vi "Main Loop.vi"(8 "error in (no error)":errorcluster, 10 "Chart Notifier":refnum<notifier>, 11 "Message Queues":T7) -> (0 "error out":errorcluster)   [LabVIEW 2018, in "D-O Module.lvlib" / "D-O Module Engine.lvlib"]
uses:
  D-O Module Engine.lvlib
  All Message Queues.ctl
  support/Message Queue/Message Cluster.ctl
  State Cluster.ctl
  State Enum.ctl
  Valve Clusters.ctl
  D-O Module Settings Cluster.ctl
  D-O Device Settings Cluster.ctl
  VICI Electronic Actuator/VICI Electronic Actuator Settings.ctl
  D-O Module Display.ctl
  <vilib>/Platform/TimedLoop/XDataNode/timing_clust.ctl
  <vilib>/Platform/TimedLoop/XDataNode/nitl_modes.ctl
  <vilib>/Platform/TimedLoop/XDataNode/wakeup.ctl
  Tag VIs/Tag FGV Operation Enum.ctl
  support/Message Queue/Enqueue Message (Single).vi
  <vilib>/Platform/TimedLoop/XDataNode/XDataNode.xnode
  support/Message Queue/Message Queue.lvlib
  <vilib>/Platform/TimedLoop/XDataNode/XDNodeRunTimeDep.lvlib
  D-O Module.lvlib
  Shared Variables/Dynamic Shared Variables.lvlib
  support/Command Log VIs/Command Logging.lvlib
  DIO Valve/VICI Electronic Actuator.lvlib
  support/Support Library.lvlib
panel:
  out "D-O Settings.Output Channel Names":string[](array[string])
  in  "?":T1={"State"=enum."Idle", "Start Time"=timestamp(0 s since 1904-01-01), "Current Time"=timestamp(0 s since 1904-01-01), "First Iteration"=FALSE, "Process Name"="", "Output Error"=FALSE, "Log Started"=FALSE, "Cycle Period"=50.0, "Configuration"={"Valve Settings"={"D-O Settings"={"DAQmx Task Name"="", "Output Channel"=0, "Output Channel Names"=[]}, "VICI Electronic Actuator"={"VISA resource name"="", "Mode"=enum."Two Positions With Stops", "Simulated"=FALSE}}, "Valve Type"=enum."Digital Output Valve", "Time On (Sec)"=0.0, "Time Off (Sec)"=0.0, "Run?"=FALSE}, "Data"={"D-O State"=enum."Off"}} {"Configuration"."Valve Settings"."D-O Settings"."Output Channel" items=["Choose a Channel"]}
  out "Period (s)":dbl format="%_4g"
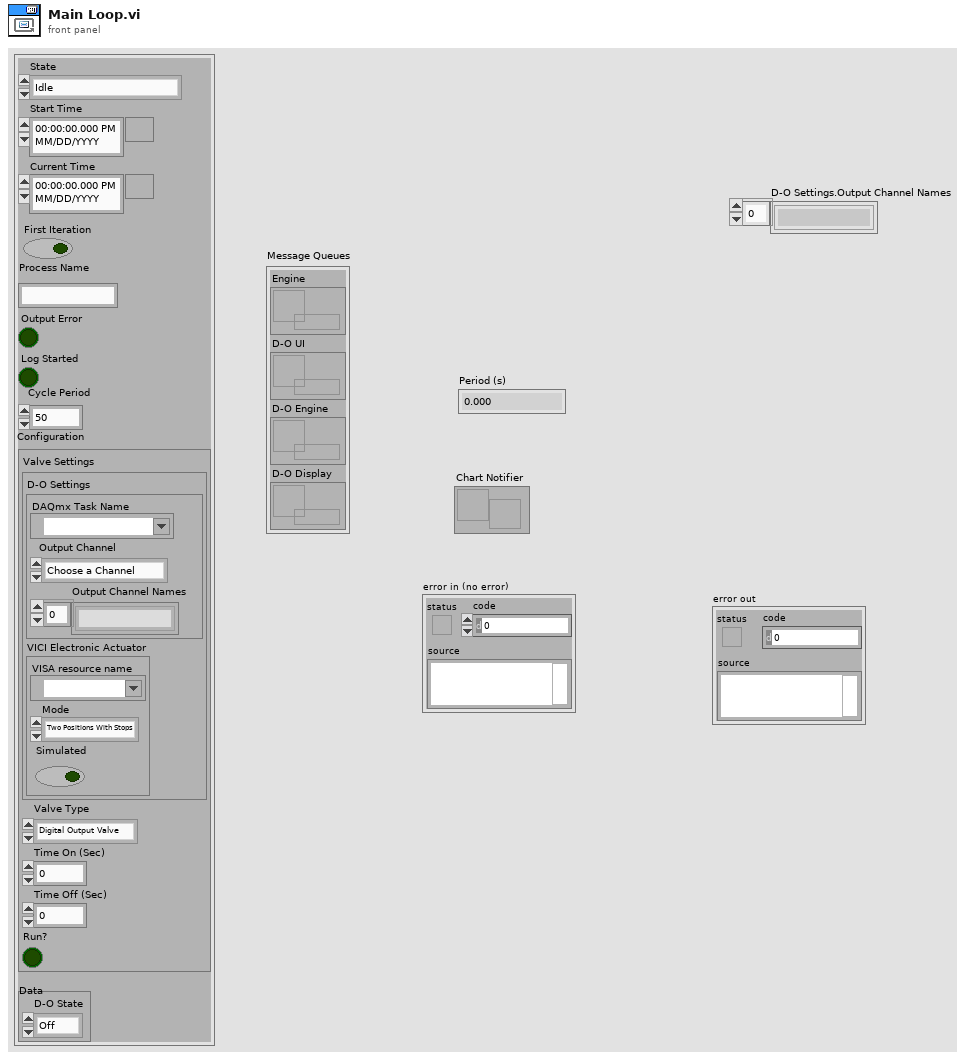
[diagram p1: front panel]
types:
  T1 = typedef "D-O Module.lvlib/D-O Module Engine.lvlib/State Cluster.ctl" = cluster{"State":T2, "Start Time":timestamp, "Current Time":timestamp, "First Iteration":bool, "Process Name":string, "Output Error":bool, "Log Started":bool, "Cycle Period":dbl, "Configuration":T3, "Data":cluster{"D-O State":enum16{"Off", "On", "Not Initialized"}}}
  T2 = typedef "D-O Module.lvlib/D-O Module Engine.lvlib/State Enum.ctl" = enum16{"Measuring", "Idle", "Paused"}
  T3 = typedef "D-O Module.lvlib/Valve Clusters.ctl" = cluster{"Valve Settings":T4, "Valve Type":enum16{"Default", "Digital Output Valve", "VICI Electronic Actuator"}, "Time On (Sec)":dbl, "Time Off (Sec)":dbl, "Run?":bool}
  T4 = typedef "D-O Module.lvlib/D-O Module Settings Cluster.ctl" = cluster{"D-O Settings":T5, "VICI Electronic Actuator":T6}
  T5 = typedef "D-O Module.lvlib/D-O Device Settings Cluster.ctl" = cluster{"DAQmx Task Name":refnum<k21>, "Output Channel":u16, "Output Channel Names":string[]}
  T6 = typedef "VICI Electronic Actuator.lvlib/VICI Electronic Actuator Settings.ctl" = cluster{"VISA resource name":refnum<visa-resource-name>, "Mode":enum16{"Two Positions With Stops", "Two Positions Without Stops", "Mutiposition"}, "Simulated":bool}
  T7 = typedef "D-O Module.lvlib/All Message Queues.ctl" = cluster{"Engine":refnum<queue>, "D-O UI":refnum<queue>, "D-O Engine":refnum<queue>, "D-O Display":refnum<queue>}
  T8 = typedef "D-O Module.lvlib/D-O Module Display.ctl" = cluster{"D-O State ":u16, "Cycle Period":dbl}
  T9 = typedef "XDNodeRunTimeDep.lvlib/timing_clust.ctl" = cluster{"Expected End [f-1]":u64, "Actual End [f-1]":u64, "Finished Late? [f-1]":bool, "Expected End [i-1]":u64, "Actual End [i-1]":u64, "Finished Late? [i-1]":bool, "Expected Start [i]":u64, "Actual Start [i]":u64, "Expected Start [f]":u64, "Actual Start [f]":u64, "Source Name":string, "Structure Name":string, "Period":i64, "Deadline":i64, "Offset":i64, "Start":i64, "Priority":i32, "Timeout":i32, "Mode":T10, "Wakeup Reason":T11, "Error":errorcluster, "Source Type":string, "Secondary Source Type":string, "Global End Time":u64, "Global Start Time":u64, "Frame Duration":u64, "Iteration Duration":u64, "Assigned CPU":i32, "I/O Scan Engine Mode":u32}
  T10 = typedef "XDNodeRunTimeDep.lvlib/nitl_modes.ctl" = enum32{"No Change", "Process missed periods, maintain original phase", "Discard missed periods, maintain original phase", "Process missed periods, ignore original phase", "Discard missed periods, ignore original phase"}
  T11 = typedef "XDNodeRunTimeDep.lvlib/wakeup.ctl" = enum32{"Normal", "Aborted", "Asynchronous wakeup", "Timing source error", "Timed loop error", "Timeout"}
  T12 = cluster{"enable? (F)":bool, "name":string, "alarm on":bool, "priority":u32, "ack type":enum16{"Auto", "User", "None", "Each Occurrence"}, "area":string, "description":string, "log? (T)":bool}
  T13 = typedef "Tag FGV Operation Enum.ctl" = enum16{"Init", "Set Notification Queue", "Create Tag", "Commit", "Write Tag (Numeric)", "Write Tag (Boolean)", "Read All Tags", "Read One Tag", "Delete Tag Category", "Set Alarm Parameters (Numeric)", "Set Alarm Parameters (Boolean)", "Enable All Alarms", "Disable All Alarms", "Delete All Tags", "Read Alarms", "Ack Alarm", "Read Alarm Parameters (Numeric)", "Read Alarm Parameters (Boolean)"}
  T14 = enum32{"u32BitField", "bool", "double", "string", "int8", "uint8", "int16", "uint16", "int32", "uint32", "int64", "uint64", "single", "double waveform", "int16 waveform", "array of boolean", "array of int8", "array of uint8", "array of int16", "array of uint16", "array of int32", "array of uint32", "array of int64", "array of uint64", "array of single", "array of double", "array of double waveform", "array of int16 waveform", "array of string", "variant", "timestamp", "fixed point", "custom"}
  T15 = enum16{"Default", "Digital Output Valve", "VICI Electronic Actuator"}
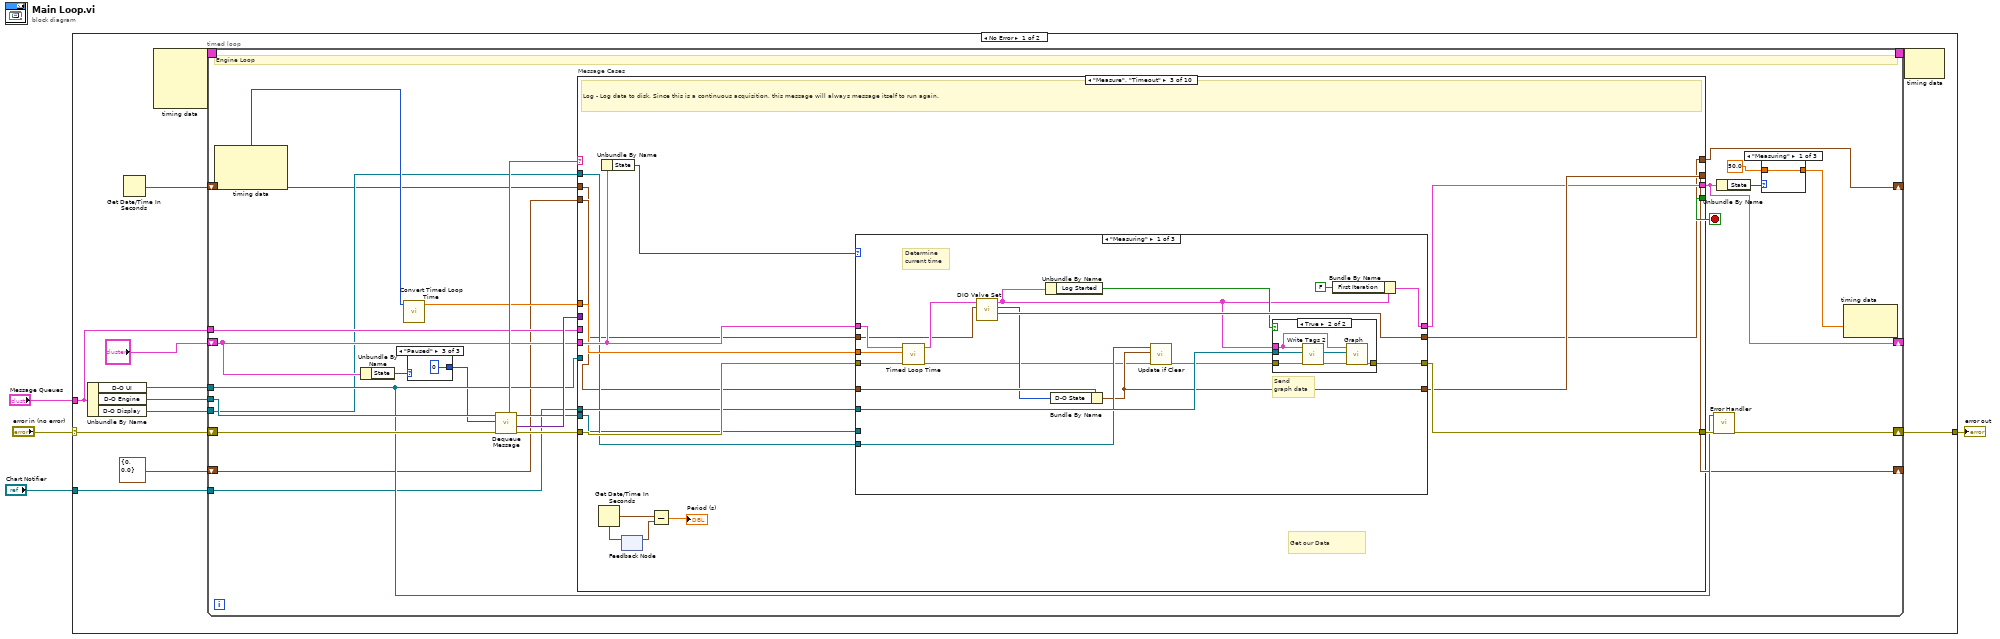
[diagram p0: block diagram]
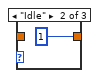
[diagram p2: hidden frame]
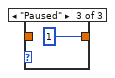
[diagram p3: hidden frame]
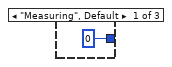
[diagram p4: hidden frame]
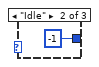
[diagram p5: hidden frame]
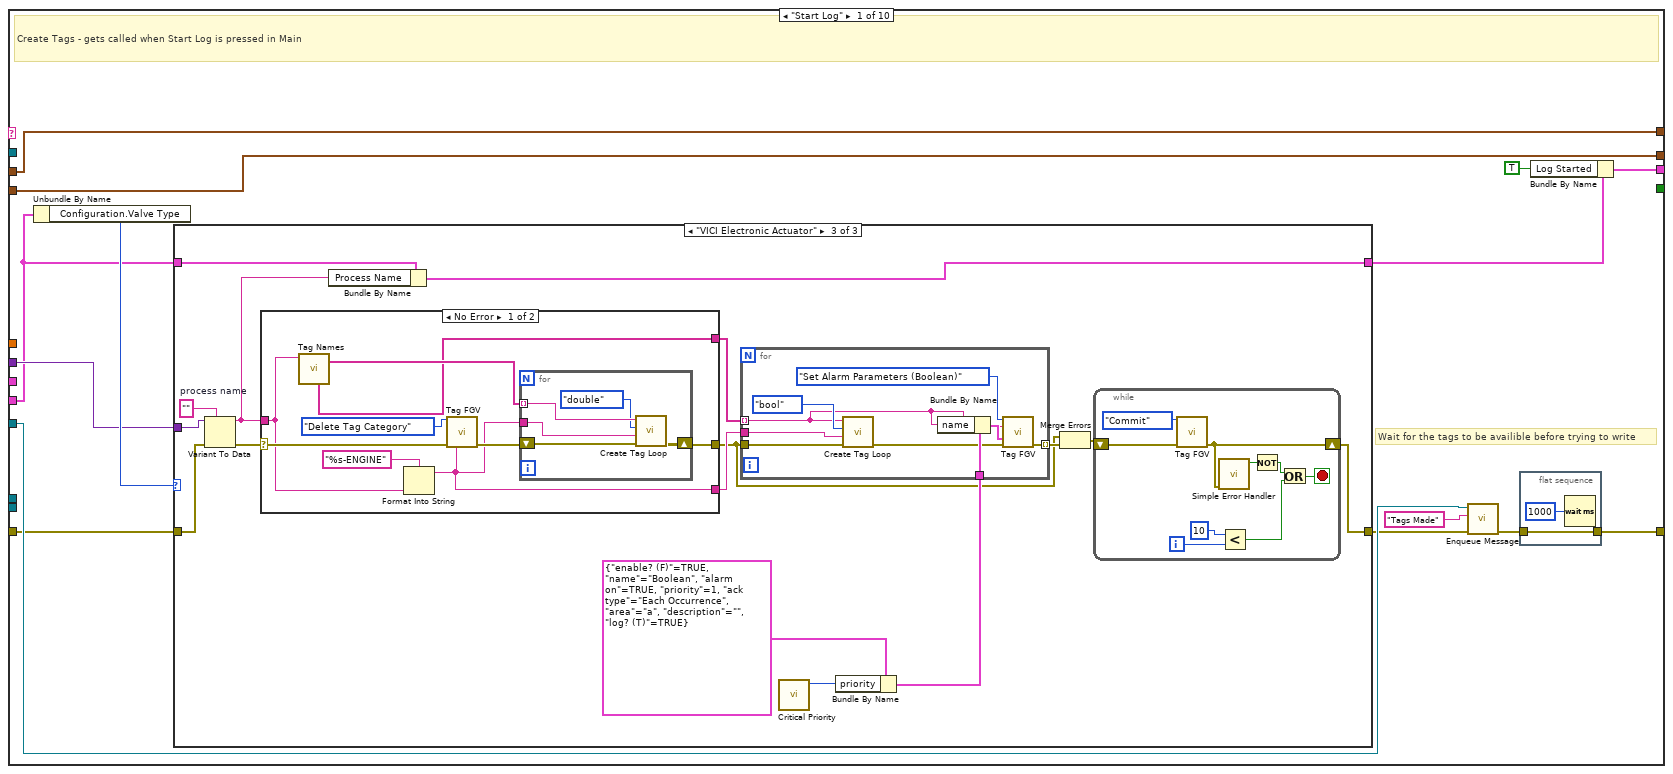
[diagram p6: hidden frame]
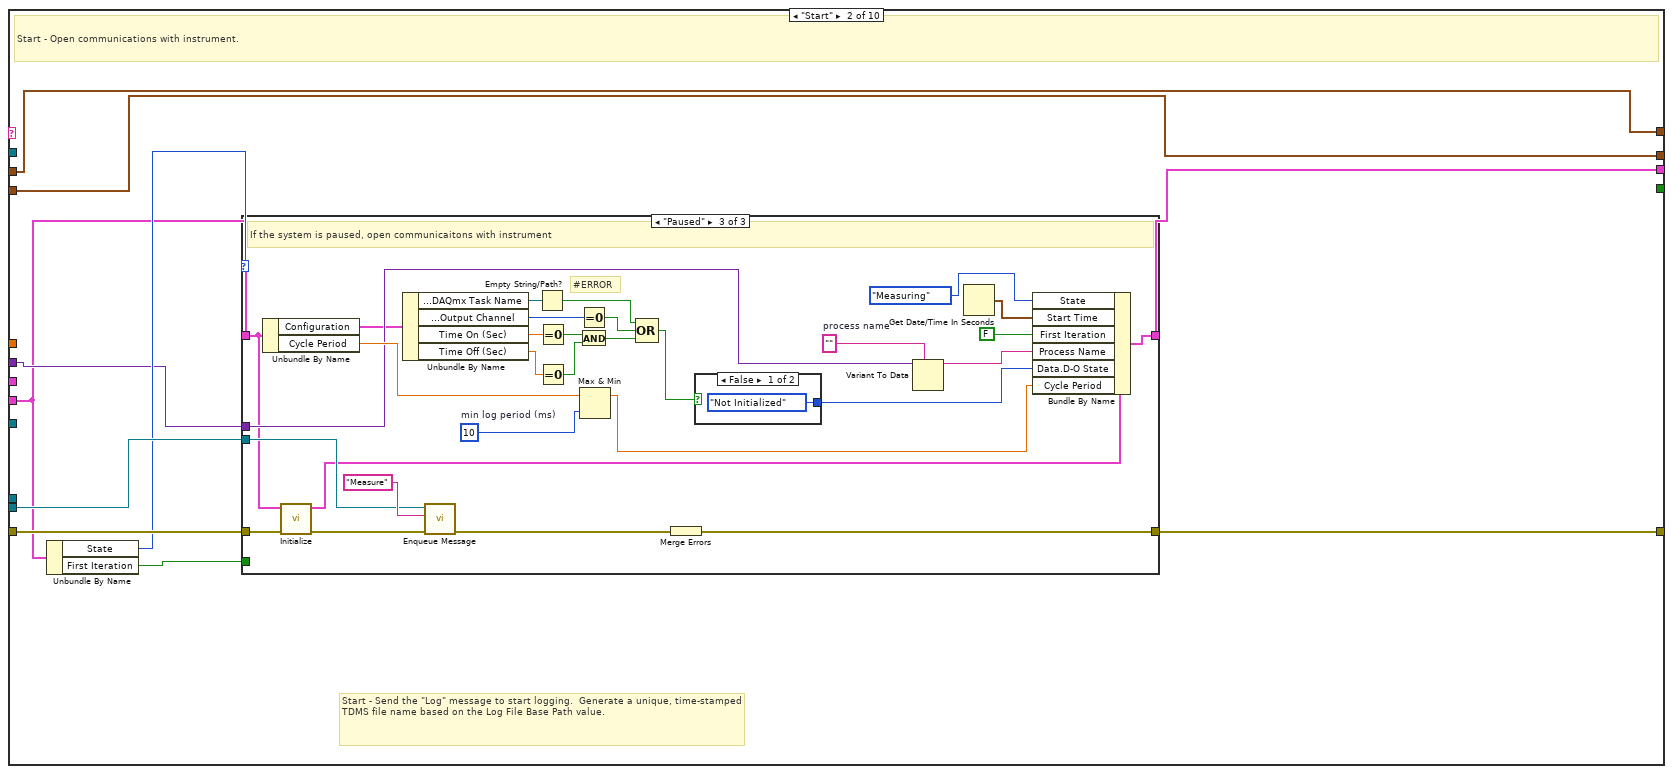
[diagram p10: hidden frame]
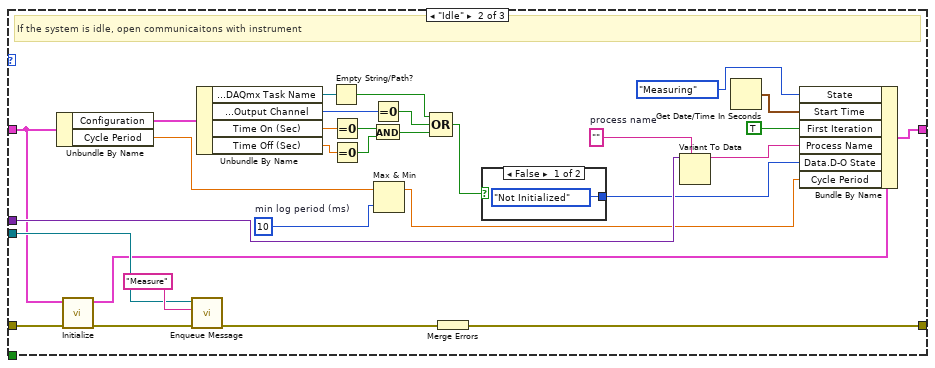
[diagram p12: hidden frame]
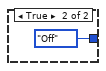
[diagram p13: hidden frame]
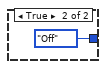
[diagram p14: hidden frame]
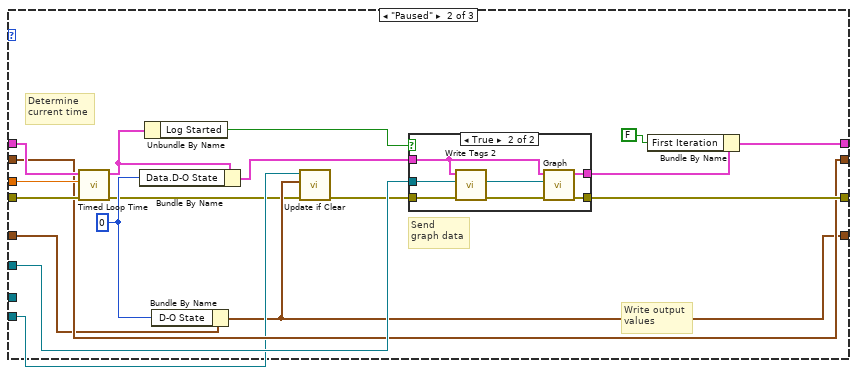
[diagram p16: hidden frame]
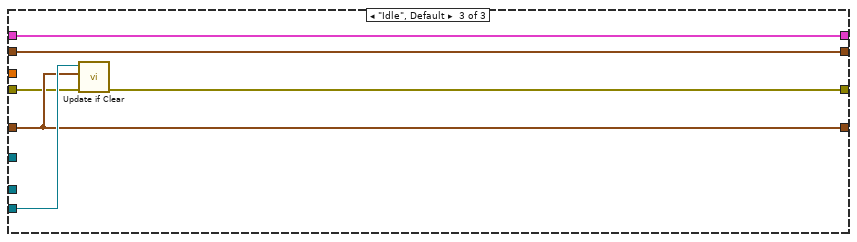
[diagram p18: hidden frame]
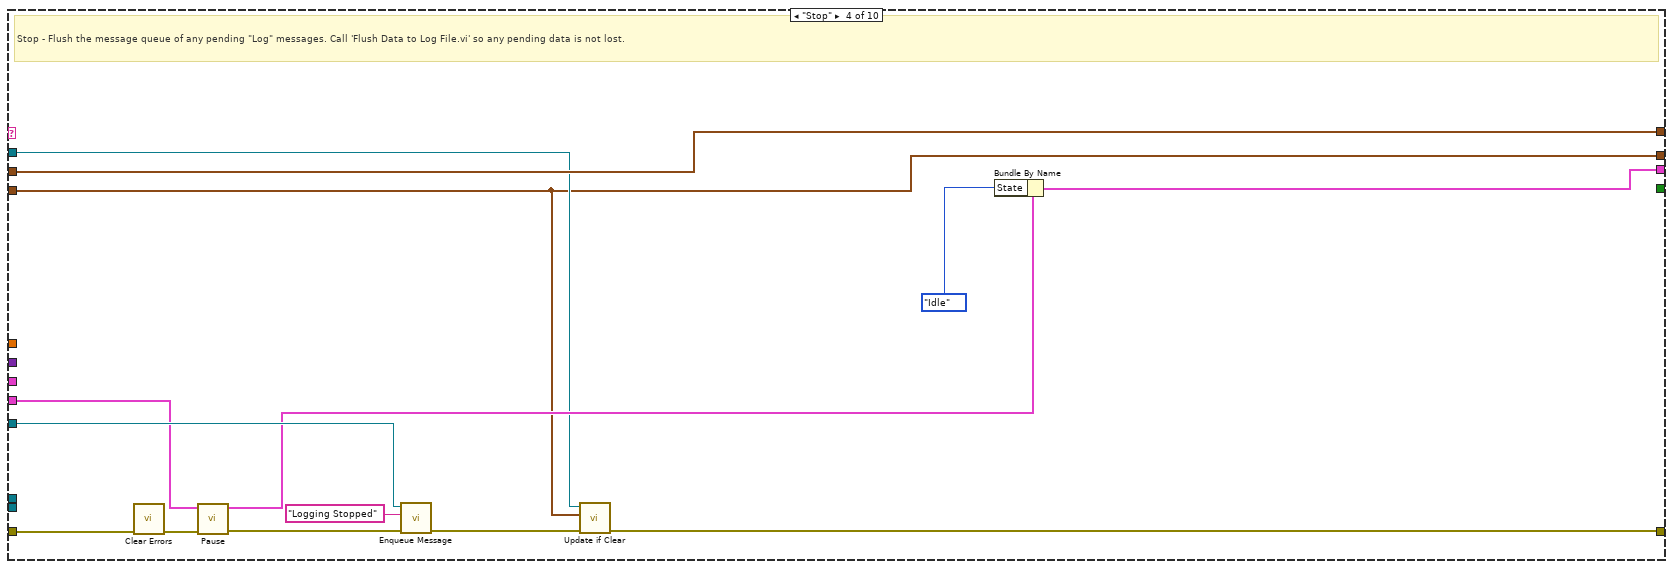
[diagram p19: hidden frame]
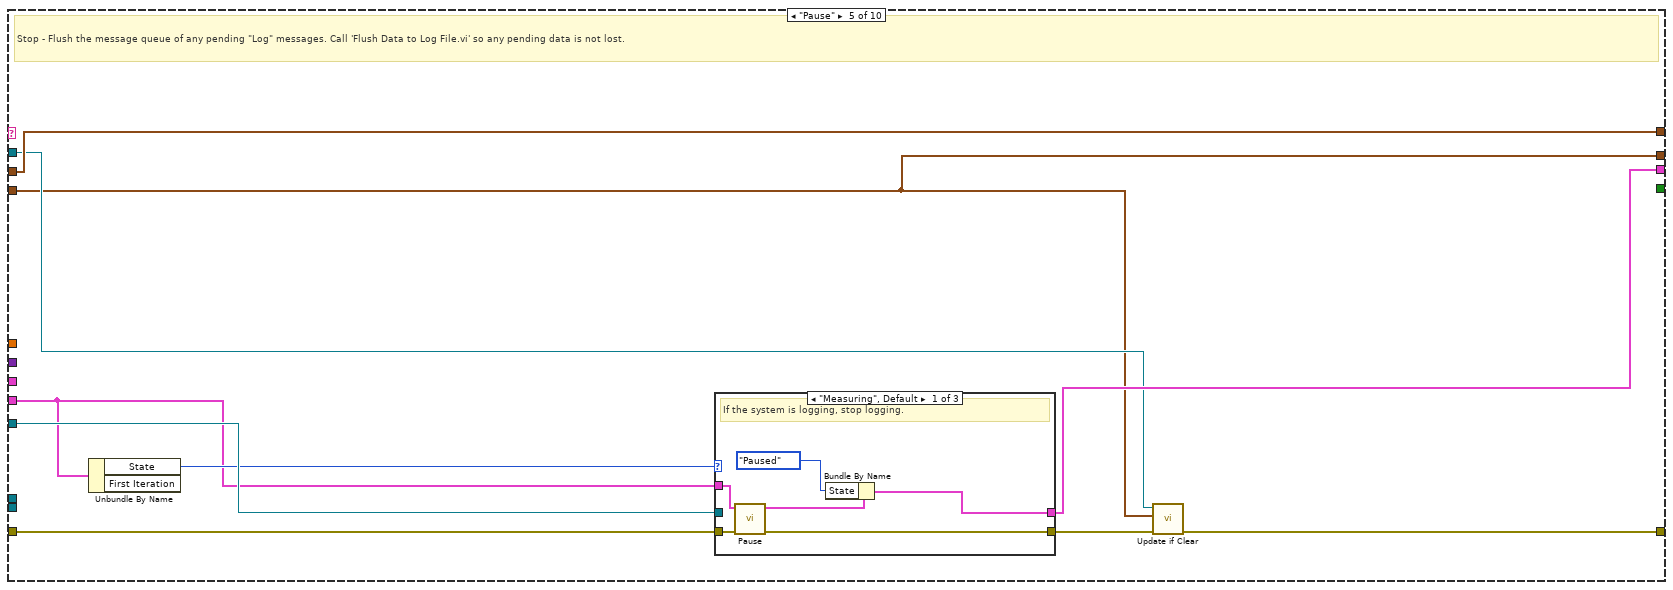
[diagram p20: hidden frame]
diagram:
  n1 = case shown="No Error" "error in (no error)" {
    selector: "error in (no error)" -> [w15 w357]
    tunnel: "Message Queues" -> [w11 _]
    tunnel: [w16 w357] -> w3
    tunnel: "Chart Notifier" -> [w9 _]
    frame No Error {
      n2 = Unbundle By Name(w11) -> ("D-O UI"=w14:refnum<queue>, "D-O Engine"=w10:refnum<queue>, "D-O Display"=w8:refnum<queue>)
      n3 = Get Date/Time In Seconds() -> (seconds since 1Jan1904=w5:timestamp)
      n4 = node-c288() -> (w13:T9)  [unwired: 4 in]
      n5 = timed-loop {
        tunnel: w10 -> [w36]
        shift-right: [w20] -> _
        shift-left: "?" -> [w32]
        shift-right: [w34] -> w16
        shift-left: w15 -> [w41]
        tunnel: w14 -> [w33]
        timing: w13 -> [_]
        timing-out: [_] -> w12
        tunnel: w11 -> [w25]
        tunnel: w9 -> [w24]
        tunnel: w8 -> [w23]
        shift-right: [w22] -> _
        shift-left: T8 {"D-O State "=0, "Cycle Period"=0.0} ("PM Display") -> [w21]
        shift-right: [w17] -> _
        shift-left: w5 -> [w18]
        stop <- w42 stop-if-true
        # "Engine Loop"
        n6 = node-c288() -> (w27:i64)  [unwired: 1 in, 2 out]
        n7 = Unbundle By Name(w32) -> ("State"=w31:T2)
        n8 = call "Convert Timed Loop Time.vi"("Actual Start [i]"=w27) -> ("ET since start (s)"=w26:dbl)  [unwired: 10 in]
        n9 = case shown="\"Paused\"" w31 {
          tunnel: [0 ("timeout in ms (-1)") -1 ("timeout in ms (-1)") 0 ("timeout in ms (-1)")] -> w30
          frame "Measuring", Default {
          }
          frame "Idle" {
          }
          frame "Paused" {
          }
        }
        n10 = call "Dequeue Message.vi"("error in (no error)"=w41, "timeout in ms (-1)"=w30, "Message Queue"=w36) -> ("error out"=w40:errorcluster, "Message Data"=w38:variant, "Message"=w39:string, "dup Message Queue"=w37:refnum<queue>)  [unwired: 5 in]
        n11 = case "Message Cases" shown="\"Measure\", \"Timeout\"" w39 {
          selector: w39 -> [_ _ _ _ _ _ _ _ _ w344]
          tunnel: w37 -> [_ w131 w202 _ _ _ w324 _ _ _]
          tunnel: w40 -> [w60 w130 w212 w282 w290 w317 w327 w335 w343 _]
          tunnel: [w54 w132 w213 w271 w285 w314 w329 w334 w342 w345] -> w35
          tunnel: w32 -> [w58 w127 w211 w276 w289 w315 w320 w332 w340 w353]
          tunnel: [w62 w124 w201 w283 w292 w312 w320 w332 w338 w353] -> w20
          tunnel: [_ _ _ _ _ _ TRUE _ _ _] -> w42
          tunnel: w38 -> [w59 w128 _ _ _ w318 _ _ _ _]
          tunnel: w33 -> [w64 _ _ w284 w294 _ w328 _ _ _]
          tunnel: w26 -> [_ _ w210 _ _ _ _ _ _ _]
          tunnel: w25 -> [_ _ _ _ _ _ _ _ _ _]
          tunnel: w24 -> [_ _ w206 _ _ _ _ _ _ _]
          tunnel: w23 -> [_ _ w205 w274 w288 _ _ _ _ _]
          tunnel: w21 -> [w67 w126 w204 w273 w287 w316 w321 w333 w341 w354]
          tunnel: [w67 w126 w203 w273 w287 w316 w321 w333 w341 w354] -> w22
          tunnel: w18 -> [w63 w123 w200 w281 w291 w313 w319 w331 w336 w352]
          tunnel: [w63 w123 w199 w281 w291 w313 w319 w331 w336 w352] -> w17
          frame "Start Log" {
            # "Wait for the tags to be availible before trying to write"
            # "Create Tags - gets called when Start Log is pressed in Main"
            n12 = Unbundle By Name(w58) -> ("Configuration.Valve Type"=w61:T15)
            n13 = case shown="\"VICI Electronic Actuator\"" w61 {
              tunnel: w60 -> [w70 w73 w79]
              tunnel: w59 -> [_ _ w78]
              tunnel: w58 -> [w71 w72 w77]
              tunnel: [w71 w72 w76] -> w57
              tunnel: [w70 w73 w75] -> w56
              frame "Default", Default {
              }
              frame "Digital Output Valve" {
              }
              frame "VICI Electronic Actuator" {
                w89 = ""  # process name
                n14 = Variant To Data(error in=w79, type=w89, Variant=w78) -> (data=w87:string, error out=w88:errorcluster)
                n15 = case shown="No Error" w88 {
                  selector: w88 -> [w113 w122]
                  tunnel: [w116 w122] -> w74
                  tunnel: w87 -> [w110 _]
                  tunnel: [w111 _] -> w83
                  tunnel: [w108 _] -> w82
                  frame No Error {
                    n16 = call "Tag Names.vi"("Process Name"=w110) -> ("All Boolean Tags"=w108:string[], "All  Numeric Tags"=w109:string[])  [unwired: 8 in, 1 out]
                    n17 = Format Into String(format string="%s-ENGINE", w110) -> (resulting string=w111:string)  [unwired: 2 in, 1 out]
                    n18 = call "Tag FGV.vi"("Operation"=Tag_FGV_Operation_Enum."Delete Tag Category", "error in (no error)"=w113, "Tag Category"=w111) -> ("error out"=w112:errorcluster)  [unwired: 5 in, 7 out]
                    n19 = for {
                      shift-right: [w121] -> w116
                      shift-left: w112 -> [w120]
                      tunnel: w111 -> [w117]
                      tunnel: w109 -> [w119] mode=indexing
                      n20 = call "Create Tag Loop.vi"("error in (no error)"=w120, "Tag Category"=w117, "data type"=T14."double", "Tag Name"=w119) -> ("error out"=w121:errorcluster)  [unwired: 7 in]
                    }
                  }
                  frame Error {
                  }
                }
                n21 = Bundle By Name(cluster=w77, "Process Name"=w87) -> (w76:T1)
                n22 = call "Critical Priority.vi"() -> ("critical priority"=w85:i32)  [unwired: 11 in]
                n23 = Bundle By Name(cluster=T12 {"enable? (F)"=TRUE, "name"="Boolean", "alarm on"=TRUE, "priority"=1, "ack type"=enum."Each Occurrence", "area"="a", "description"="", "log? (T)"=TRUE} ("Boolean alarm settings"), "priority"=w85) -> (w84:T12)
                n24 = for {
                  tunnel: w84 -> [w107]
                  tunnel: [w106] -> w81 mode=indexing
                  tunnel: w82 -> [w99] mode=indexing
                  tunnel: w83 -> [w100]
                  tunnel: w74 -> [w103]
                  n25 = call "Create Tag Loop.vi"("error in (no error)"=w103, "Tag Category"=w100, "data type"=T14."bool", "Tag Name"=w99) -> ("error out"=w101:errorcluster)  [unwired: 7 in]
                  n26 = Bundle By Name(cluster=w107, "name"=w99) -> (w105:T12)
                  n27 = call "Tag FGV.vi"("Operation"=Tag_FGV_Operation_Enum."Set Alarm Parameters (Boolean)", "Tag Name"=w99, "Data"=w105, "error in (no error)"=w101) -> ("error out"=w106:errorcluster)  [unwired: 4 in, 7 out]
                }
                n28 = Merge Errors(w74, w81) -> (w80:errorcluster)
                n29 = while {
                  shift-right: [w96] -> w75
                  shift-left: w80 -> [w97]
                  i -> [w94]
                  stop <- w90 stop-if-true
                  n30 = call "Tag FGV.vi"("Operation"=Tag_FGV_Operation_Enum."Commit", "error in (no error)"=w97) -> ("error out"=w96:errorcluster)  [unwired: 6 in, 7 out]
                  n31 = call <vilib>:"Simple Error Handler.vi"("error in (no error)"=w96) -> ("error?"=w95:bool)  [unwired: 4 in, 4 out]
                  n32 = Less?(x=10, y=w94) -> (x < y?=w91:bool)
                  n33 = Not(x=w95) -> (.not. x?=w92:bool)
                  n34 = Or(x=w92, y=w91) -> (x .or. y?=w90:bool)
                }
              }
            }
            n35 = call-poly "Enqueue Message.vi"("error in (no error)"=w56, "Message"="Tags Made", "Message Queue"=w64) -> ("error out"=w55:errorcluster)  [unwired: 7 in, 1 out]
            n36 = flat-sequence {
              tunnel: [w68] -> w54
              tunnel: w55 -> [w68]
              frame #0 {
                n37 = Wait (ms)(milliseconds to wait=u32 1000) -> ()  [unwired: 1 out]
              }
            }
            n38 = Bundle By Name(cluster=w57, "Log Started"=TRUE) -> (w62:T1)
          }
          frame "Start" {
            # "Start - Send the \"Log\" message to start logging.  Generate a unique, time-stamped TDMS file name based on the Log File Base Path value."
            # "Start - Open communications with instrument."
            n39 = Unbundle By Name(w127) -> ("State"=w129:T2, "First Iteration"=w125:bool)
            n40 = case shown="\"Paused\"" w129 {
              tunnel: [w133 w164 w196] -> w132
              tunnel: w131 -> [_ w156 w188]
              tunnel: w130 -> [w133 w138 w171]
              tunnel: w127 -> [w134 w139 w169]
              tunnel: [w134 w162 w194] -> w124
              tunnel: w128 -> [_ w153 w185]
              tunnel: w125 -> [_ _ _]
              frame "Measuring", Default {
                # "The system is already running. Ignore the \"Start\" message."
              }
              frame "Idle" {
                w154 = ""  # process name
                w159 = 10  # min log period (ms)
                # "If the system is idle, open communicaitons with instrument"
                n41 = Unbundle By Name(w139) -> ("Configuration"=w150:T3, "Cycle Period"=w158:dbl)
                n42 = call "Initialize.vi"("error in (no error)"=w138, "State in"=w139) -> ("error out"=w137:errorcluster, "State out"=w136:T1)  [unwired: 7 in, 1 out]
                n43 = call-poly "Enqueue Message.vi"("error in (no error)"=w137, "Message"="Measure", "Message Queue"=w156) -> ("error out"=w160:errorcluster)  [unwired: 7 in, 1 out]
                n44 = Unbundle By Name(w150) -> ("Valve Settings.D-O Settings.DAQmx Task Name"=w149:refnum<k21>, "Valve Settings.D-O Settings.Output Channel"=w140:u16, "Time On (Sec)"=w144:dbl, "Time Off (Sec)"=w147:dbl)
                n45 = Empty String/Path?(string/path=w149) -> (empty?=w148:bool)
                n46 = Equal To 0?(x=w144) -> (x = 0?=w146:bool)
                n47 = Equal To 0?(x=w147) -> (x = 0?=w145:bool)
                n48 = Equal To 0?(x=w140) -> (x = 0?=w143:bool)
                n49 = And(x=w146, y=w145) -> (x .and. y?=w142:bool)
                n50 = Max & Min(x=w158, y=w159) -> (max(x,y)=w135:dbl)  [unwired: 1 out]
                n51 = Compound Arithmetic op=OR(w148, w143, w142) -> (w141:bool)
                n52 = Merge Errors(w160) -> (w164:errorcluster)
                n53 = case shown="False" w141 {
                  tunnel: [enum16{"Off", "On", "Not Initialized"}."Not Initialized" ("Pump On?") enum16{"Off", "On", "Not Initialized"}."Off" ("Pump On?")] -> w151
                  frame False {
                  }
                  frame True {
                  }
                }
                n54 = Variant To Data(type=w154, Variant=w153) -> (data=w152:string)  [unwired: 1 in, 1 out]
                n55 = Get Date/Time In Seconds() -> (seconds since 1Jan1904=w157:timestamp)
                n56 = Bundle By Name(cluster=w136, "State"=State_Enum."Measuring", "Start Time"=w157, "First Iteration"=TRUE, "Process Name"=w152, "Data.D-O State"=w151, "Cycle Period"=w135) -> (w162:T1)
              }
              frame "Paused" {
                w186 = ""  # process name
                w191 = 10  # min log period (ms)
                # "#ERROR"
                # "If the system is paused, open communicaitons with instrument"
                n57 = Unbundle By Name(w169) -> ("Configuration"=w182:T3, "Cycle Period"=w190:dbl)
                n58 = call "Initialize.vi"("error in (no error)"=w171, "State in"=w169) -> ("error out"=w170:errorcluster, "State out"=w168:T1)  [unwired: 7 in, 1 out]
                n59 = Unbundle By Name(w182) -> ("Valve Settings.D-O Settings.DAQmx Task Name"=w181:refnum<k21>, "Valve Settings.D-O Settings.Output Channel"=w172:u16, "Time On (Sec)"=w176:dbl, "Time Off (Sec)"=w179:dbl)
                n60 = call-poly "Enqueue Message.vi"("error in (no error)"=w170, "Message"="Measure", "Message Queue"=w188) -> ("error out"=w192:errorcluster)  [unwired: 7 in, 1 out]
                n61 = Empty String/Path?(string/path=w181) -> (empty?=w180:bool)
                n62 = Equal To 0?(x=w176) -> (x = 0?=w178:bool)
                n63 = Equal To 0?(x=w179) -> (x = 0?=w177:bool)
                n64 = Equal To 0?(x=w172) -> (x = 0?=w175:bool)
                n65 = And(x=w178, y=w177) -> (x .and. y?=w174:bool)
                n66 = Max & Min(x=w190, y=w191) -> (max(x,y)=w167:dbl)  [unwired: 1 out]
                n67 = Compound Arithmetic op=OR(w180, w175, w174) -> (w173:bool)
                n68 = Merge Errors(w192) -> (w196:errorcluster)
                n69 = case shown="False" w173 {
                  tunnel: [enum16{"Off", "On", "Not Initialized"}."Not Initialized" ("Pump On?") enum16{"Off", "On", "Not Initialized"}."Off" ("Pump On?")] -> w183
                  frame False {
                  }
                  frame True {
                  }
                }
                n70 = Variant To Data(type=w186, Variant=w185) -> (data=w184:string)  [unwired: 1 in, 1 out]
                n71 = Get Date/Time In Seconds() -> (seconds since 1Jan1904=w189:timestamp)
                n72 = Bundle By Name(cluster=w168, "State"=State_Enum."Measuring", "Start Time"=w189, "First Iteration"=FALSE, "Process Name"=w184, "Data.D-O State"=w183, "Cycle Period"=w167) -> (w194:T1)
              }
            }
          }
          frame "Measure", "Timeout" {
            # "Get our Data"
            # "Log - Log data to disk. Since this is a continuous acquisition, this message will always message itself to run again."
            n73 = Get Date/Time In Seconds() -> (seconds since 1Jan1904=w208:timestamp)
            n74 = Unbundle By Name(w211) -> ("State"=w214:T2)
            n75 = feedback-in #1(w208) -> ()
            n76 = feedback #1() -> (w209:timestamp)  [unwired: 1 in]
            n77 = Subtract(x=w208, y=w209) -> (x-y=→"Period (s)":dbl)
            n78 = case shown="\"Measuring\"" w214 {
              tunnel: w212 -> [w231 w255 w266]
              tunnel: w211 -> [w226 w248 w270]
              tunnel: [w232 w256 w265] -> w213
              tunnel: [w229 w252 w270] -> w201
              tunnel: w210 -> [w230 w254 _]
              tunnel: w206 -> [w227 w250 _]
              tunnel: w205 -> [w220 w242 w268]
              tunnel: w204 -> [w223 w244 w267]
              tunnel: [w219 w241 w267] -> w203
              tunnel: w202 -> [_ _ _]
              tunnel: w200 -> [w221 w245 w269]
              tunnel: [w224 w245 w269] -> w199
              frame "Measuring" {
                # "Determine\ncurrent time"
                # "Send\ngraph data"
                n79 = call "Timed Loop Time.vi"("error in (no error)"=w231, "ET since start (s)"=w230, "State in"=w226) -> ("error out"=w218:errorcluster, "State out"=w225:T1)  [unwired: 7 in]
                n80 = call "DIO Valve Set.vi"("current time"=w221, "State in"=w225) -> ("time"=w224:timestamp, "Numeric"=w222:i32, "State out"=w215:T1)  [unwired: 7 in]
                n81 = Unbundle By Name(w215) -> ("Log Started"=w216:bool)
                n82 = Bundle By Name(cluster=w223, "D-O State"=w222) -> (w219:T8)
                n83 = call "Update if Clear.vi"("error in (no error)"=w218, "Message Data"=w219, "Queue in"=w220) -> ("error out"=w217:errorcluster)  [unwired: 8 in]
                n84 = case shown="True" w216 {
                  tunnel: [w233 w238] -> w232
                  tunnel: w227 -> [_ w237]
                  tunnel: w215 -> [_ w236]
                  tunnel: w217 -> [w233 w235]
                  frame False {
                  }
                  frame True {
                    n85 = call "Write Tags 2.vi"("error in (no error)"=w235, "State in"=w236) -> ("error out"=w234:errorcluster)  [unwired: 9 in]
                    n86 = call "Graph.vi"("error in (no error)"=w234, "notifier out"=w237, "State in"=w236) -> ("error out"=w238:errorcluster)  [unwired: 7 in, 1 out]
                  }
                }
                n87 = Bundle By Name(cluster=w215, "First Iteration"=FALSE) -> (w229:T1)
              }
              frame "Paused" {
                w243 = 0
                # "Determine\ncurrent time"
                # "Send\ngraph data"
                # "Write output\nvalues"
                n88 = call "Timed Loop Time.vi"("error in (no error)"=w255, "ET since start (s)"=w254, "State in"=w248) -> ("error out"=w240:errorcluster, "State out"=w247:T1)  [unwired: 7 in]
                n89 = Bundle By Name(cluster=w247, "Data.D-O State"=w243) -> (w246:T1)
                n90 = Unbundle By Name(w247) -> ("Log Started"=w249:bool)
                n91 = Bundle By Name(cluster=w244, "D-O State"=w243) -> (w241:T8)
                n92 = call "Update if Clear.vi"("error in (no error)"=w240, "Message Data"=w241, "Queue in"=w242) -> ("error out"=w239:errorcluster)  [unwired: 8 in]
                n93 = case shown="True" w249 {
                  tunnel: [w257 w264] -> w256
                  tunnel: [w258 w263] -> w253
                  tunnel: w250 -> [_ w262]
                  tunnel: w246 -> [w258 w261]
                  tunnel: w239 -> [w257 w260]
                  frame False {
                  }
                  frame True {
                    n94 = call "Write Tags 2.vi"("error in (no error)"=w260, "State in"=w261) -> ("error out"=w259:errorcluster)  [unwired: 9 in]
                    n95 = call "Graph.vi"("error in (no error)"=w259, "notifier out"=w262, "State in"=w261) -> ("error out"=w264:errorcluster, "State out"=w263:T1)  [unwired: 7 in]
                  }
                }
                n96 = Bundle By Name(cluster=w253, "First Iteration"=FALSE) -> (w252:T1)
              }
              frame "Idle", Default {
                n97 = call "Update if Clear.vi"("error in (no error)"=w266, "Message Data"=w267, "Queue in"=w268) -> ("error out"=w265:errorcluster)  [unwired: 8 in]
              }
            }
          }
          frame "Stop" {
            # "Stop - Flush the message queue of any pending \"Log\" messages. Call 'Flush Data to Log File.vi' so any pending data is not lost."
            n98 = call <vilib>:"Clear Errors.vi"("error in (no error)"=w282) -> ("error out"=w278:errorcluster)  [unwired: 5 in, 1 out]
            n99 = call "Pause.vi"("error in (no error)"=w278, "State in"=w276) -> ("error out"=w277:errorcluster, "State out"=w275:T1)  [unwired: 8 in]
            n100 = call-poly "Enqueue Message.vi"("error in (no error)"=w277, "Message"="Logging Stopped", "Message Queue"=w284) -> ("error out"=w272:errorcluster)  [unwired: 7 in, 1 out]
            n101 = call "Update if Clear.vi"("error in (no error)"=w272, "Message Data"=w273, "Queue in"=w274) -> ("error out"=w271:errorcluster)  [unwired: 8 in]
            n102 = Bundle By Name(cluster=w275, "State"=State_Enum."Idle") -> (w283:T1)
          }
          frame "Pause" {
            # "Stop - Flush the message queue of any pending \"Log\" messages. Call 'Flush Data to Log File.vi' so any pending data is not lost."
            n103 = Unbundle By Name(w289) -> ("State"=w293:T2)  [unwired: 1 out]
            n104 = case shown="\"Measuring\", Default" w293 {
              tunnel: [w295 w301 w308] -> w286
              tunnel: w290 -> [w299 w301 w308]
              tunnel: w294 -> [_ _ _]
              tunnel: w289 -> [w296 w302 w306]
              tunnel: [w297 w303 w305] -> w292
              frame "Measuring", Default {
                # "If the system is logging, stop logging."
                n105 = call "Pause.vi"("error in (no error)"=w299, "State in"=w296) -> ("error out"=w295:errorcluster, "State out"=w298:T1)  [unwired: 8 in]
                n106 = Bundle By Name(cluster=w298, "State"=State_Enum."Paused") -> (w297:T1)
              }
              frame "Idle" {
                # "The system is already idle. Ignore the \"Stop\" message."
                n107 = Bundle By Name(cluster=w302, "State"=State_Enum."Paused") -> (w303:T1)
              }
              frame "Paused" {
                n108 = Bundle By Name(cluster=w306, "State"=State_Enum."Paused") -> (w305:T1)
              }
            }
            n109 = call "Update if Clear.vi"("error in (no error)"=w286, "Message Data"=w287, "Queue in"=w288) -> ("error out"=w285:errorcluster)  [unwired: 8 in]
          }
          frame "Update Settings" {
            # "New settings are available, update the current ones stored in the shift register with the settings sent as part of the message"
            n110 = Variant To Data(error in=w317, type=T3 {"Valve Settings"={"D-O Settings"={"DAQmx Task Name"="", "Output Channel"=0, "Output Channel Names"=[]}, "VICI Electronic Actuator"={"VISA resource name"="", "Mode"=enum."Two Positions With Stops", "Simulated"=FALSE}}, "Valve Type"=enum."Digital Output Valve", "Time On (Sec)"=0.0, "Time Off (Sec)"=0.0, "Run?"=FALSE} ("Configuration"), Variant=w318) -> (data=w311:T3, error out=w314:errorcluster)
            n111 = Bundle By Name(cluster=w315, "Configuration"=w311) -> (w312:T1)
            n112 = Unbundle By Name(w311) -> ("Valve Settings.D-O Settings.Output Channel Names"=→"D-O Settings.Output Channel Names":string[])
          }
          frame "Exit" {
            # "Release the Logging queue reference"
            # "Don't check the error out. The UI message queue may have already been released."
            # "Stop the VI"
            # "Exit - Send the Exit message to the UI Message Handler.  Call 'Flush Data to Log File.vi' so any pending data is not lost."
            n113 = Release Queue(queue=w324, error in (no error)=w327) -> (error out=w323:errorcluster)  [unwired: 1 in, 2 out]
            n114 = call-poly "Enqueue Message.vi"("Priority Message? (F)"=TRUE, "Message"="Exit", "Message Queue"=w328) -> ("error out"=w322:errorcluster)  [unwired: 7 in, 1 out]
            n115 = call <vilib>:"Clear Errors.vi"("error in (no error)"=w322) -> ()  [unwired: 5 in, 2 out]
            n116 = Merge Errors(w323) -> (w329:errorcluster)
          }
          frame "---Copy This Frame---" {
            # "Duplicate this frame when creating new messages.  Change this comment in the duplicated frame to describe this message."
            n117 = Merge Errors(w335) -> (w334:errorcluster)
          }
          frame "Initialize" {
            # "Duplicate this frame when creating new messages.  Change this comment in the duplicated frame to describe this message."
            n118 = Bundle By Name(cluster=w340, "Log Started"=FALSE, "First Iteration"=TRUE) -> (w338:T1)
            n119 = Merge Errors(w343) -> (w342:errorcluster)
          }
          frame Default {
            # "'Default' case only runs if there is a message that isn't defined in any of the other cases.  Output a programming error."
            n120 = Concatenate Strings("The invalid message string " ("string"), w344, " was received in D-O Engine." ("string")) -> (w346:string)
            n121 = Bundle By Name(cluster=errorcluster {"status"=TRUE, "code"=1, "source"=""} ("error constant"), "source"=w346) -> (w345:errorcluster)
            n122 = Concatenate Strings("DO Module: " ("text"), w344) -> (w350:string)
            n123 = call "Write to Log File.vi"("error in"=w345, "text"=w350) -> ()  [unwired: 9 in, 1 out]
          }
        }
        n124 = call "Error Handler.vi"("error in (no error)"=w35, "Message Queue"=w33) -> ("dup error in"=w34:errorcluster)  [unwired: 8 in, 1 out]
        n125 = Unbundle By Name(w20) -> ("State"=w29:T2)
        n126 = case shown="\"Measuring\"" w29 {
          tunnel: [w43 1 1] -> w28
          tunnel: 50.0 ("Cycle Period") -> [w43 _ _]
          frame "Measuring" {
          }
          frame "Idle" {
          }
          frame "Paused" {
          }
        }
        n127 = node-c288(w28) -> ()  [unwired: 1 in, 1 out]
      }
      n128 = node-c288(w12) -> ()  [unwired: 1 out]
    }
    frame Error {
    }
  }
  "error out" <- w3
